vi "check status.vi"(8 "error in (no error)":errorcluster) -> (0 "error out":errorcluster, 2 "status":bool)   [LabVIEW 2016, in "FPGA Resource Manager.lvlib"]
uses:
  FPGA Resource Manager.lvlib
  global constants.vi
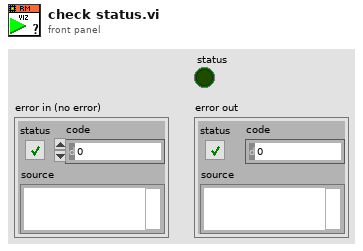
[diagram p1: front panel]
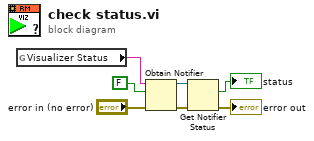
[diagram p0: block diagram]
diagram:
  n1 = global read "global constants.vi" "Visualizer Status"() -> (w7:string)
  n2 = Obtain Notifier(name (unnamed)=w7, notification data type=FALSE, error in (no error)="error in (no error)") -> (notifier out=w5:refnum<notifier>, error out=w4:errorcluster)  [unwired: 1 in, 1 out]
  n3 = Get Notifier Status(notifier=w5, error in (no error)=w4) -> (current notification=→"status":bool, error out=→"error out":errorcluster)  [unwired: 3 out]
